vi "AssertEquals.vi"(5 "Expected":variant, 7 "Message (\"\")":string, 8 "error in (no error)":errorcluster, 10 "Actual":variant) -> (0 "error out":errorcluster, 2 "Result":bool)   [LabVIEW 2019, in "Assertion.lvlib"]
doc: "Asserts that two variables are equal. Does nothing if an error occurred before this node runs. Returns an error if the assertion failed. Optionally adds a message to the error message if the assertion failed."
uses:
  Assertion.lvlib
  Constraint/IsEqual/IsEqual.lvclass
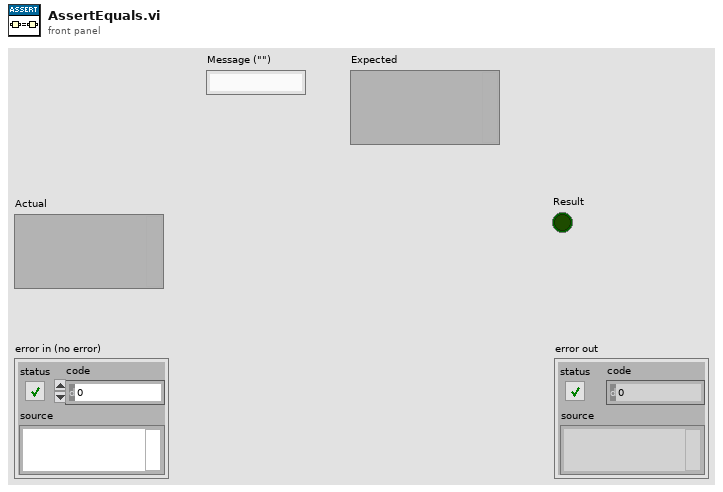
[diagram p1: front panel]
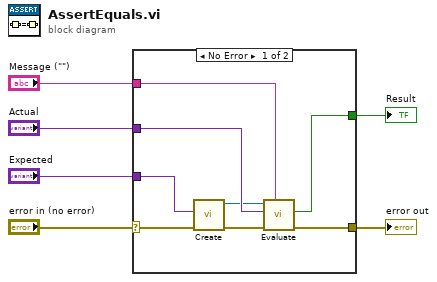
[diagram p0: block diagram]
diagram:
  n1 = case shown="No Error" "error in (no error)" {
    selector: "error in (no error)" -> [w10 w15]
    tunnel: "Actual" -> [w14 _]
    tunnel: [w13 _] -> w5
    tunnel: [w12 w15] -> w4
    tunnel: "Message (\"\")" -> [w11 _]
    tunnel: "Expected" -> [w7 _]
    frame No Error {
      n2 = call "Create.vi"("error in (no error)"=w10, "Expected"=w7) -> ("error out"=w9:errorcluster, "IsEqual"=w8:refnum<class "IsEqual.lvclass">)  [unwired: 8 in]
      n3 = call-dynamic "Evaluate.vi"("Message (\"\")"=w11, "error in (no error)"=w9, "Actual"=w14, "Constraint in"=w8) -> ("error out"=w12:errorcluster, "Result"=w13:bool)  [unwired: 5 in, 1 out]
    }
    frame Error {
    }
  }
  "error out" <- w4
  "Result" <- w5
